vi "8.10.-Momento h7.vi"(1 "n30/n12/n21/n03":dbl[](array[numeric])) -> (0 "M7":dbl)   [LabVIEW 2020]
panel:
  # "Visión Artificial - Momentos Invariantes de Hu\nDiego Cervantes Rodríguez\ndicer0.com"
  # "M7 = ((3*n21-n03)*(n30+n12)*((n30+n12)^2 -3*(n21+n03)^2))+((n30-3*n12)*(n21+n03)*(3*(n30+n12)^2 -(n21+n03)^2))"
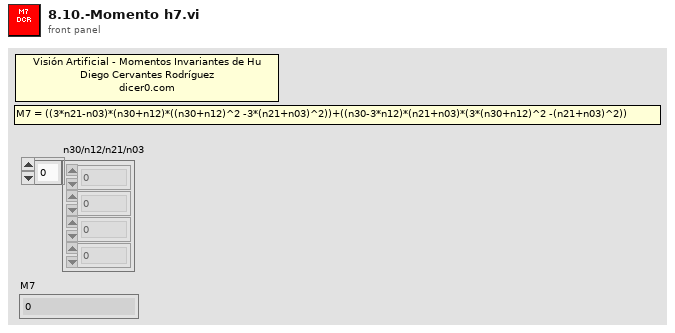
[diagram p1: front panel]
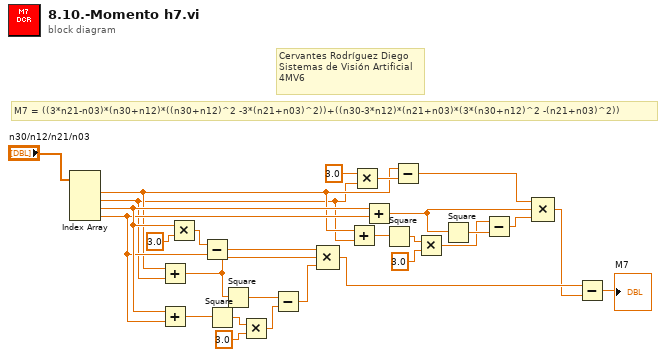
[diagram p0: block diagram]
diagram:
  # "M7 = ((3*n21-n03)*(n30+n12)*((n30+n12)^2 -3*(n21+n03)^2))+((n30-3*n12)*(n21+n03)*(3*(n30+n12)^2 -(n21+n03)^2))"
  # "Cervantes Rodríguez Diego\nSistemas de Visión Artificial\n4MV6"
  n1 = Index Array(array="n30/n12/n21/n03") -> (element #1=w16:dbl, element #2=w15:dbl, element #3=w18:dbl, element #4=w17:dbl)  [unwired: 4 in]
  n2 = Add(x=w16, y=w15) -> (x+y=w22:dbl)
  n3 = Add(x=w18, y=w17) -> (x+y=w26:dbl)
  n4 = Multiply(x=w18, y=3.0) -> (x*y=w27:dbl)
  n5 = Subtract(x=w27, y=w17) -> (x-y=w20:dbl)
  n6 = Square(x=w26) -> (x^2=w25:dbl)
  n7 = Square(x=w22) -> (x^2=w24:dbl)
  n8 = Multiply(x=w25, y=3.0) -> (x*y=w23:dbl)
  n9 = Subtract(x=w24, y=w23) -> (x-y=w21:dbl)
  n10 = Compound Arithmetic op=MULTIPLY(w20, w22, w21) -> (w6:dbl)
  n11 = Add(x=w16, y=w15) -> (x+y=w14:dbl)
  n12 = Multiply(x=3.0, y=w15) -> (x*y=w19:dbl)
  n13 = Add(x=w18, y=w17) -> (x+y=w9:dbl)
  n14 = Square(x=w14) -> (x^2=w12:dbl)
  n15 = Subtract(x=w16, y=w19) -> (x-y=w8:dbl)
  n16 = Multiply(x=w12, y=3.0) -> (x*y=w10:dbl)
  n17 = Square(x=w9) -> (x^2=w11:dbl)
  n18 = Subtract(x=w10, y=w11) -> (x-y=w7:dbl)
  n19 = Compound Arithmetic op=MULTIPLY(w8, w9, w7) -> (w5:dbl)
  n20 = Subtract(x=w6, y=w5) -> (x-y=→"M7":dbl)
